vi "Visible Caption.vi"(8 "error in (no error)":errorcluster, 10 "caption":enum8{"hide", "show"}(ring), 11 "GObject in":refnum<vi>) -> (0 "error out":errorcluster, 1 "was caption visible?":enum8{"hide", "show"}(ring), 2 "has caption?":bool, 3 "GObject out":refnum<vi>)   [LabVIEW 2019, in "Builtins.lvlib"]
doc: "Shows or hides the caption on controls.\n\nCreated by: Ryan Pacini"
uses:
  Builtins.lvlib
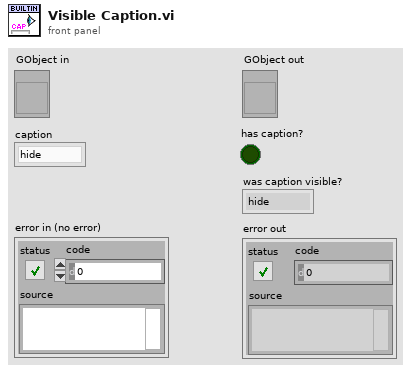
[diagram p1: front panel]
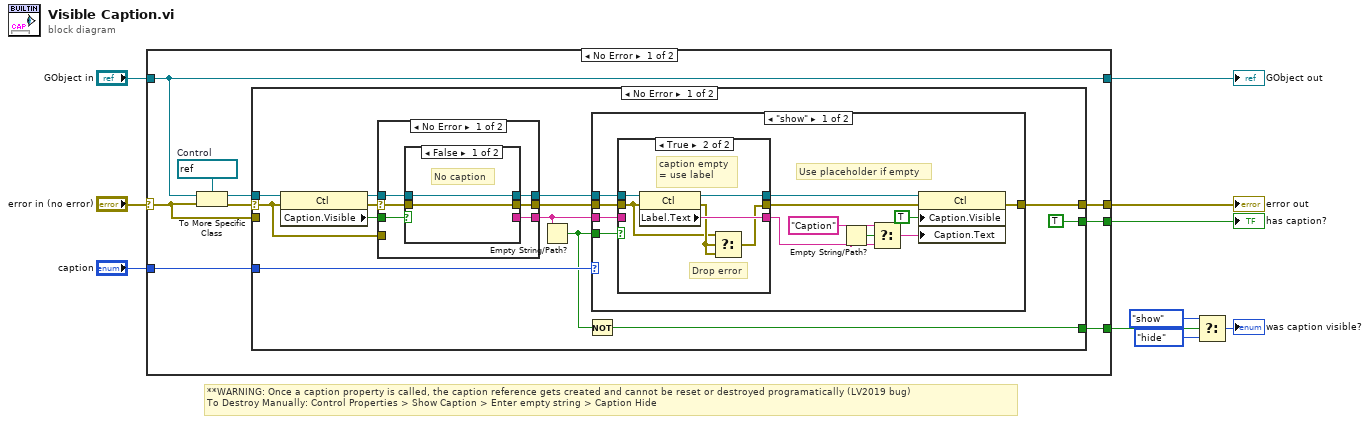
[diagram p0: block diagram]
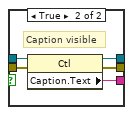
[diagram p2: hidden frame]
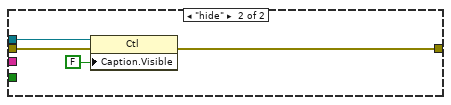
[diagram p5: hidden frame]
diagram:
  # "**WARNING: Once a caption property is called, the caption reference gets created and cannot be reset or destroyed programatically (LV2019 bug)\nTo Destroy Manually: Control Properties > Show Caption > Enter empty string > Caption Hide"
  n1 = case shown="No Error" "error in (no error)" {
    selector: "error in (no error)" -> [w11 w74]
    tunnel: "caption" -> [w12 _]
    tunnel: [w19 _] -> w5
    tunnel: [w18 w74] -> w4
    tunnel: "GObject in" -> [w17 w75]
    tunnel: [w17 w75] -> w2
    tunnel: [w16 _] -> w1
    frame No Error {
      w13 = refnum<vi> refnum  # Control
      n2 = To More Specific Class(target class=w13, reference=w17, error in=w11) -> (specific class reference=w14:refnum<vi>, error out=w15:errorcluster)
      n3 = case shown="No Error" w15 {
        selector: w15 -> [w23 _]
        tunnel: [w20 _] -> w19
        tunnel: [w29 w73] -> w18
        tunnel: [TRUE _] -> w16
        tunnel: w14 -> [w31 _]
        tunnel: w12 -> [w30 _]
        tunnel: w11 -> [_ w73]
        frame No Error {
          n4 = property class="Ctl"(reference=w31, error in=w23) -> (reference out=w28:refnum<vi>, error out=w27:errorcluster, "Caption.Visible"=w26:bool)
          n5 = case shown="No Error" w27 {
            selector: w27 -> [w37 _]
            tunnel: w28 -> [w38 w47]
            tunnel: w26 -> [w36 _]
            tunnel: [w35 _] -> w25
            tunnel: [w34 w47] -> w24
            tunnel: w23 -> [_ w46]
            tunnel: [w33 w46] -> w22
            frame No Error {
              n6 = case shown="False" w36 {
                tunnel: w38 -> [w40 w45]
                tunnel: w37 -> [w39 w44]
                tunnel: [_ w43] -> w35
                tunnel: [w40 w42] -> w34
                tunnel: [w39 w41] -> w33
                frame False {
                  # "No caption"
                }
                frame True {
                  # "Caption visible"
                  n7 = property class="Ctl"(reference=w45, error in=w44) -> (reference out=w42:refnum<vi>, error out=w41:errorcluster, "Caption.Text"=w43:string)
                }
              }
            }
            frame Error {
              # "Drop caption error"
            }
          }
          n8 = Empty String/Path?(string/path=w25) -> (empty?=w21:bool)
          n9 = Not(x=w21) -> (.not. x?=w20:bool)
          n10 = case shown="\"show\"" w30 {
            tunnel: [w59 w72] -> w29
            tunnel: w24 -> [w58 w71]
            tunnel: w21 -> [w56 _]
            tunnel: w25 -> [w55 _]
            tunnel: w22 -> [w49 w69]
            frame "show" {
              # "Use placeholder if empty"
              n11 = case shown="True" w56 {
                tunnel: w58 -> [w62 w68]
                tunnel: [w62 w67] -> w57
                tunnel: [w61 w66] -> w52
                tunnel: w55 -> [w61 _]
                tunnel: w49 -> [w60 w64]
                tunnel: [w60 w63] -> w48
                frame False {
                  # "caption not empty"
                }
                frame True {
                  # "Drop error"
                  # "caption empty\n= use label"
                  n12 = property class="Ctl"(reference=w68, error in=w64) -> (reference out=w67:refnum<vi>, error out=w65:errorcluster, "Label.Text"=w66:string)
                  n13 = Select(t=w64, s=w65, f=w65) -> (s? t:f=w63:errorcluster)
                }
              }
              n14 = Empty String/Path?(string/path=w52) -> (empty?=w53:bool)
              n15 = Select(t="Caption", s=w53, f=w52) -> (s? t:f=w51:string)
              n16 = property class="Ctl"(reference=w57, error in=w48, "Caption.Visible"=TRUE, "Caption.Text"=w51) -> (error out=w59:errorcluster)  [unwired: 1 out]
            }
            frame "hide" {
              n17 = property class="Ctl"(reference=w71, error in=w69, "Caption.Visible"=FALSE) -> (error out=w72:errorcluster)  [unwired: 1 out]
            }
          }
        }
        frame Error {
        }
      }
    }
    frame Error {
    }
  }
  "error out" <- w4
  "GObject out" <- w2
  "has caption?" <- w1
  n18 = Select(t=enum8{"hide", "show"}."show" ("was inc/dec visible?"), s=w5, f=enum8{"hide", "show"}."hide" ("was inc/dec visible?")) -> (s? t:f=→"was caption visible?":enum8{"hide", "show"})
